vi "Run.vi"(8 "error in (no error)":errorcluster caption="entrée d'erreur (pas d'erreur)", 11 "ParameterGrid.lvclass":refnum<class "ParameterGrid.lvclass">) -> (0 "error out":errorcluster caption="sortie d'erreur", 2 "Data":string[][](array[string]), 3 "ParameterGrid.lvclass":refnum<class "ParameterGrid.lvclass">)   [LabVIEW 2020, in "ParameterGrid.lvclass"]
doc: "Return : Grid of parameters with a discrete number of values for each."
uses:
  ParameterGrid.lvclass
  ParameterGrid.lvclass/ParameterGrid.ctl
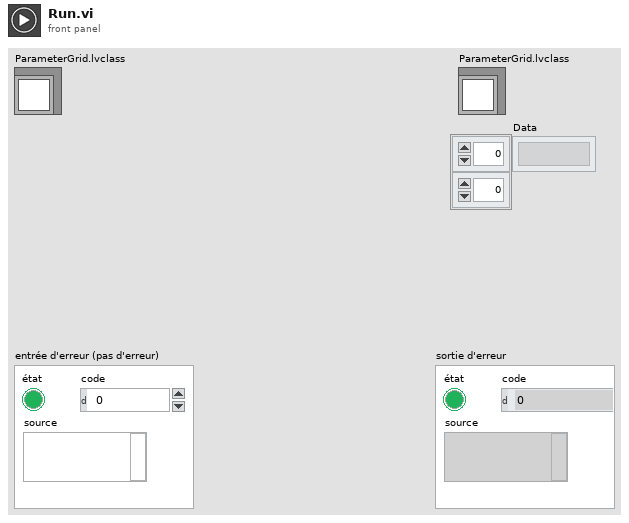
[diagram p1: front panel]
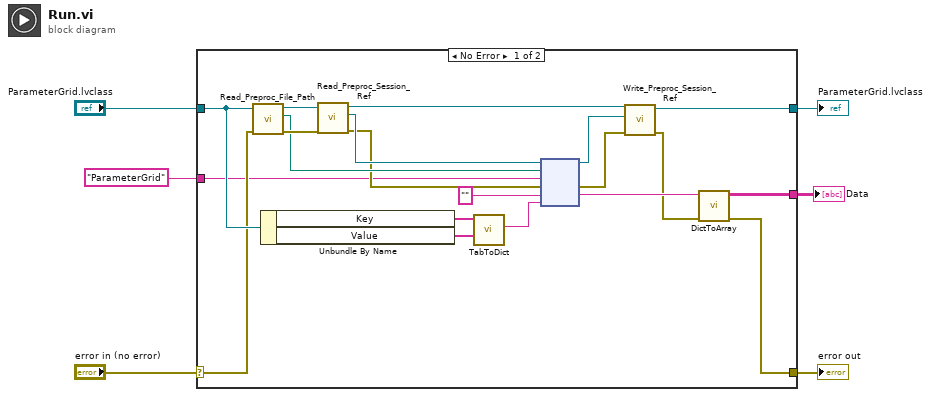
[diagram p0: block diagram]
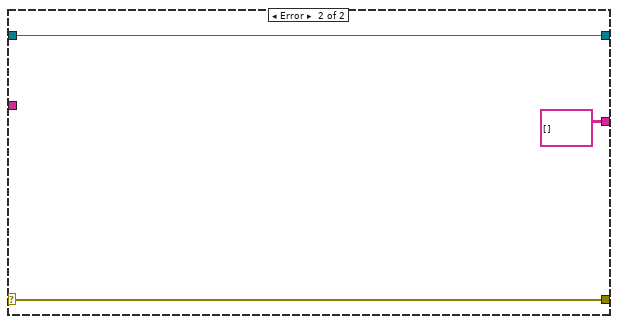
[diagram p2: hidden frame]
diagram:
  n1 = case shown="No Error" "error in (no error)" {
    selector: "error in (no error)" -> [w16 w29]
    tunnel: [w7 w29] -> w5
    tunnel: [w14 w28] -> w3
    tunnel: "ParameterGrid.lvclass" -> [w17 w28]
    tunnel: "ParameterGrid" -> [w15 _]
    tunnel: [w9 string[][] [] ("String 2DArray")] -> w1
    frame No Error {
      n2 = call-dynamic "Read_Preproc_File_Path.vi"("error in (no error)"=w16, "Python in"=w17) -> ("error out"=w25:errorcluster, "File_Path"=w24:path, "Python out"=w26:refnum<class "ParameterGrid.lvclass">)  [unwired: 7 in]
      n3 = Unbundle By Name(w17) -> ("Key"=w13:string[], "Value"=w12:string[])
      n4 = call-dynamic "Read_Preproc_Session_Ref.vi"("error in (no error)"=w25, "Python in"=w26) -> ("error out"=w22:errorcluster, "Session_ref"=w23:refnum<k35>, "Python out"=w21:refnum<class "ParameterGrid.lvclass">)  [unwired: 7 in]
      n5 = call "TabToDict.vi"("String Value"=w12, "String key"=w13) -> ("Dict with string value"=w11:string)  [unwired: 8 in, 1 out]
      n6 = node(w23, w24, w15, w22, "", w11) -> (w19:refnum<k35>, w20:errorcluster, w10:string)  [unwired: 1 in, 2 out]
      n7 = call-dynamic "Write_Preproc_Session_Ref.vi"("error in (no error)"=w20, "Session_ref"=w19, "Python in"=w21) -> ("error out"=w8:errorcluster, "Python out"=w14:refnum<class "ParameterGrid.lvclass">)  [unwired: 7 in]
      n8 = call "DictToArray.vi"("entrée d'erreur (pas d'erreur)"=w8, "Dict"=w10) -> ("sortie d'erreur"=w7:errorcluster, "String 2DArray"=w9:string[][])  [unwired: 8 in]
    }
    frame Error {
    }
  }
  "error out" <- w5
  "ParameterGrid.lvclass" <- w3
  "Data" <- w1
